vi "LSX Get Zw Travel.vi"(8 "error in (no error)":errorcluster, 9 "pdDistance":dbl, 10 "lIndex":i32, 11 "lLSID":i32) -> (0 "error out":errorcluster, 1 "pdDistance out":dbl, 3 "function return":i32)   [LabVIEW 2018, in "Tango.lvlib"]
doc: "TANGOAPI int TANGOCALL LSX_GetZwTravel (int lLSID, int lIndex, double *pdDistance);"
uses:
  Tango.lvlib
  SubVIs/Tango_DLL.dll
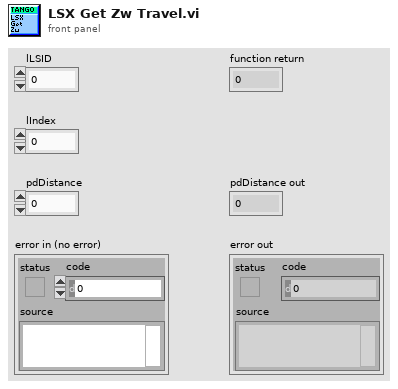
[diagram p1: front panel]
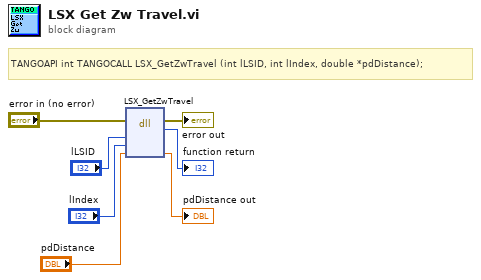
[diagram p0: block diagram]
diagram:
  # "TANGOAPI int TANGOCALL LSX_GetZwTravel (int lLSID, int lIndex, double *pdDistance);"
  n1 = dll-call lib="C:/Users/Familie/Documents/LabviewIX81/lib/TANGO Stage/SubVIs/Tango_DLL.*" fn="LSX_GetZwTravel"(error in="error in (no error)", "lLSID"="lLSID", "lIndex"="lIndex", "pdDistance"="pdDistance") -> (error out=→"error out":errorcluster, →"function return":i32, "pdDistance"=→"pdDistance out":dbl)  [unwired: 4 in, 1 out]
